vi "polynomial value (SubVI).vi"(9 "coeffs":dbl[](array[numeric]), 11 "x":dbl[](array[numeric])) -> (3 "y":dbl[](array[numeric]))   [LabVIEW 2024]
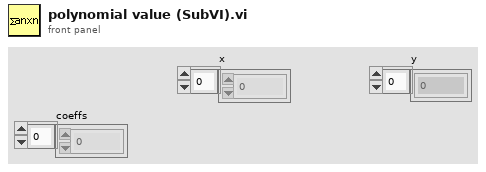
[diagram p1: front panel]
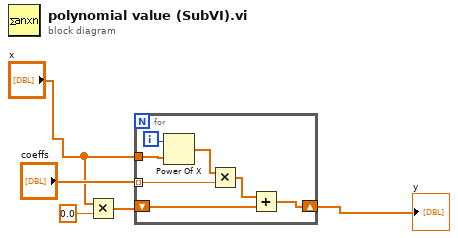
[diagram p0: block diagram]
diagram:
  n1 = Multiply(x="x", y=0.0) -> (x*y=w2:dbl[])
  n2 = for {
    tunnel: "coeffs" -> [w9] mode=indexing
    tunnel: "x" -> [w12]
    shift-right: [w6] -> w1
    shift-left: w2 -> [w7]
    i -> [w11]
    n3 = Power Of X(1:w12, 2:w11) -> (0:w10:dbl[])
    n4 = Multiply(x=w10, y=w9) -> (x*y=w8:dbl[])
    n5 = Add(x=w8, y=w7) -> (x+y=w6:dbl[])
  }
  "y" <- w1
